vi "Update Job File to new template.vi"   [LabVIEW 2019]
types:
  T1 = cluster{"Jobs No":string, "Key Value":string[]}[]
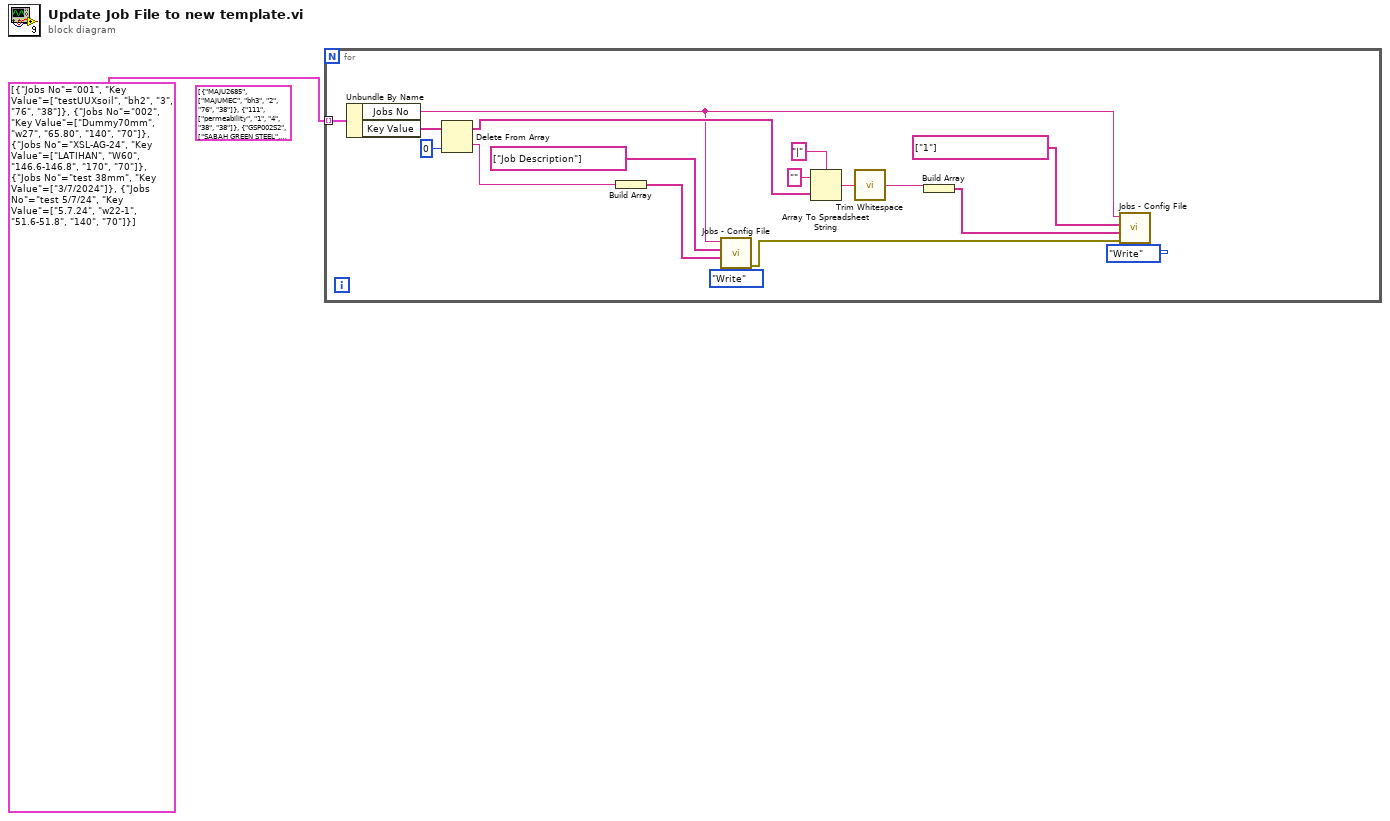
[diagram p0: block diagram]
diagram:
  (unwired) T1 [{"Jobs No"="MAJU2685", "Key Value"=["MAJUMEC", "bh3", "2", "76", "38"]}, {"Jobs No"="111", "Key Value"=["permeability", "1", "4", "38", "38"]}, {"Jobs No"="GSP002S2", "Key Value"=["SABAH GREEN STEEL", "NNO1U3", "18.50-19.00", "76", "38"]}, {"Jobs No"="GSP002S3", "Key Value"=["SABAH GREEN STEEL", "NN02U2", "12.50-13.00", "76", "38"]}] ("Value Out")
  n1 = for {
    tunnel: T1 [{"Jobs No"="001", "Key Value"=["testUUXsoil", "bh2", "3", "76", "38"]}, {"Jobs No"="002", "Key Value"=["Dummy70mm", "w27", "65.80", "140", "70"]}, {"Jobs No"="XSL-AG-24", "Key Value"=["LATIHAN", "W60", "146.6-146.8", "170", "70"]}, {"Jobs No"="test 38mm", "Key Value"=["3/7/2024"]}, {"Jobs No"="test 5/7/24", "Key Value"=["5.7.24", "w22-1", "51.6-51.8", "140", "70"]}] ("Value Out") -> [w18] mode=indexing
    n2 = Unbundle By Name(w18) -> ("Jobs No"=w5:string, "Key Value"=w14:string[])
    n3 = Delete From Array(array=w14, index=0) -> (deleted portion=w13:string, array with subset deleted=w7:string[])  [unwired: 1 in]
    n4 = Build Array(w13) -> (w15:string[])
    n5 = call "Jobs - Config File.vi"("Action"=enum16{"Write", "Read", "Read All", "Remove"}."Write", "Value"=w15, "Key Name"=string[] ["Job Description"], "Jobs No"=w5) -> ("error out"=w2:errorcluster)  [unwired: 5 in, 2 out]
    n6 = Array To Spreadsheet String(delimiter (Tab)="|", array=w7, 3:"" ("format string")) -> (spreadsheet string=w8:string)
    n7 = call <vilib>:"Trim Whitespace.vi"("string"=w8) -> ("trimmed string"=w4:string)  [unwired: 1 in]
    n8 = Build Array(w4) -> (w3:string[])
    n9 = call "Jobs - Config File.vi"("Action"=enum16{"Write", "Read", "Read All", "Remove"}."Write", "error in (no error)"=w2, "Value"=w3, "Key Name"=string[] ["1"], "Jobs No"=w5) -> ()  [unwired: 4 in, 3 out]
  }
